vi "Read Compressor Pressure.vi"() -> (1 "Solenoid Voltage":dbl, 2 "Input Voltage":dbl, 3 "Compressor current (A)":dbl)   [LabVIEW 2018]
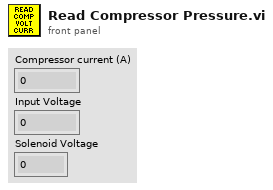
[diagram p1: front panel]
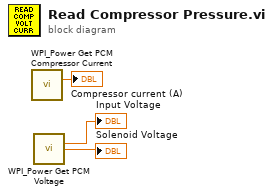
[diagram p0: block diagram]
diagram:
  n1 = call <vilib>:"WPI_Power Get PCM Compressor Current.vi"() -> ("current (A)"=→"Compressor current (A)":dbl)  [unwired: 14 in, 1 out]
  n2 = call <vilib>:"WPI_Power Get PCM Voltage.vi"() -> ("Input Voltage"=→"Input Voltage":dbl, "Solenoid Voltage"=→"Solenoid Voltage":dbl)  [unwired: 13 in, 1 out]
